vi "Get Custom SCP Command.vi"(8 "error in (no error)":errorcluster, 11 "Section Ref in":T1 format="%.0x") -> (0 "error out":errorcluster, 2 "Custom SCP Commands (str)":string[](array[string]), 3 "Section Ref out":T1 format="%.0x")   [LabVIEW 2023, in "Vires VTD System Explorer.lvlib"]
uses:
  Vires VTD System Explorer.lvlib
  <vilib>/NI VeriStand/Custom Device API/Custom Device Item Ref.ctl
  Shared/Constants.vi
  <vilib>/NI VeriStand/Custom Device Tools/Custom Device Utility Library/NI VeriStand - Search for Item by GUID.vi
  Shared/Vires VTD Shared.lvlib
  <vilib>/NI VeriStand/Custom Device Tools/Custom Device Utility Library/Custom Device Utility Library.lvlib
  <vilib>/NI VeriStand/Custom Device API/Custom Device API.lvlib
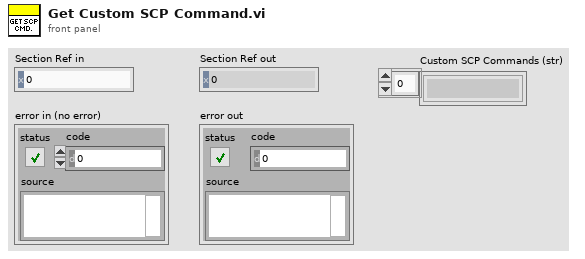
[diagram p1: front panel]
types:
  T1 = typedef "Custom Device API.lvlib/Custom Device Item Ref.ctl" = u64
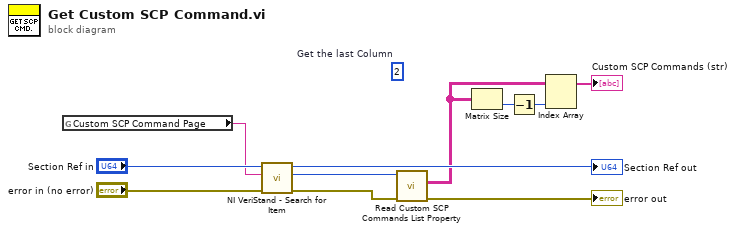
[diagram p0: block diagram]
diagram:
  (unwired) 2  # Get the last Column
  n1 = global read "Constants.vi" "Custom SCP Command Page"() -> (w9:string)
  n2 = call-poly <vilib>:"NI VeriStand - Search for Item.vi"("error in"="error in (no error)", "Item GUID"=w9, "Section Ref in"="Section Ref in") -> ("error out"=w6:errorcluster, "Item Ref"=w7:T1, "Section Ref out"=→"Section Ref out":T1)  [unwired: 5 in, 1 out]
  n3 = call "Read Custom SCP Commands List Property.vi"("error in (no error)"=w6, "Node Ptr"=w7) -> ("error out"=→"error out":errorcluster, "Custom SCP Commands List"=w2:string[][])  [unwired: 7 in, 1 out]
  n4 = Matrix Size(0:w2) -> (2:w3:i32)  [unwired: 1 out]
  n5 = Decrement(x=w3) -> (x-1=w1:i32)
  n6 = Index Array(array=w2, index (col)=w1) -> (element=→"Custom SCP Commands (str)":string[])  [unwired: 1 in]
